vi "PIDStartMotors.vi"(11 "Refnum in":refnum<k20>) -> (1 "PacketOut":u8[](array[numeric]))   [LabVIEW 2011]
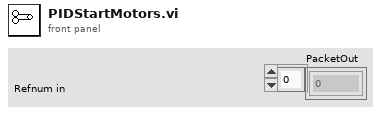
[diagram p1: front panel]
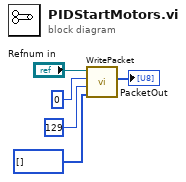
[diagram p0: block diagram]
diagram:
  n1 = call "WritePacket.vi"("Payload"=u8[] [], "Type"=u8 129, "Status"=u8 0, "Refnum in"="Refnum in") -> ("PacketOut"=→"PacketOut":u8[])  [unwired: 7 in]
